vi "AnalyzerDataToString.vi"(8 "ErrorIn":errorcluster, 11 "WebServicesData":T2) -> (0 "ErrorOut":errorcluster, 3 "String":string)   [LabVIEW 2019]
uses:
  MobileAnalyzer/mainVIs/communicateWebServicesVIs/WebServicesData.ctl
  MobileAnalyzer/mainVIs/analyzeAccelerationDataVIs/AccelerationDataFrames.ctl
  MobileAnalyzer/mainVIs/UIVIs/UIOutput.ctl
  <vilib>/wsapi/NI_WebServices.lvlib
panel:
  in  "VisualizedData":enum32{"Page 1", "Page 2"}(tab)
  out "Phases":T1(graph)
  out "Amplitudes":cluster{"f0":dbl, "df":dbl, "real part":dbl[]}[](graph)
  out "Acceleration":waveform(dbl)[](graph)
  out "Aquiring data":bool
  out "FIFO overflow":bool
  out "Analyzing data":bool
  out "AnalyzerError":errorcluster
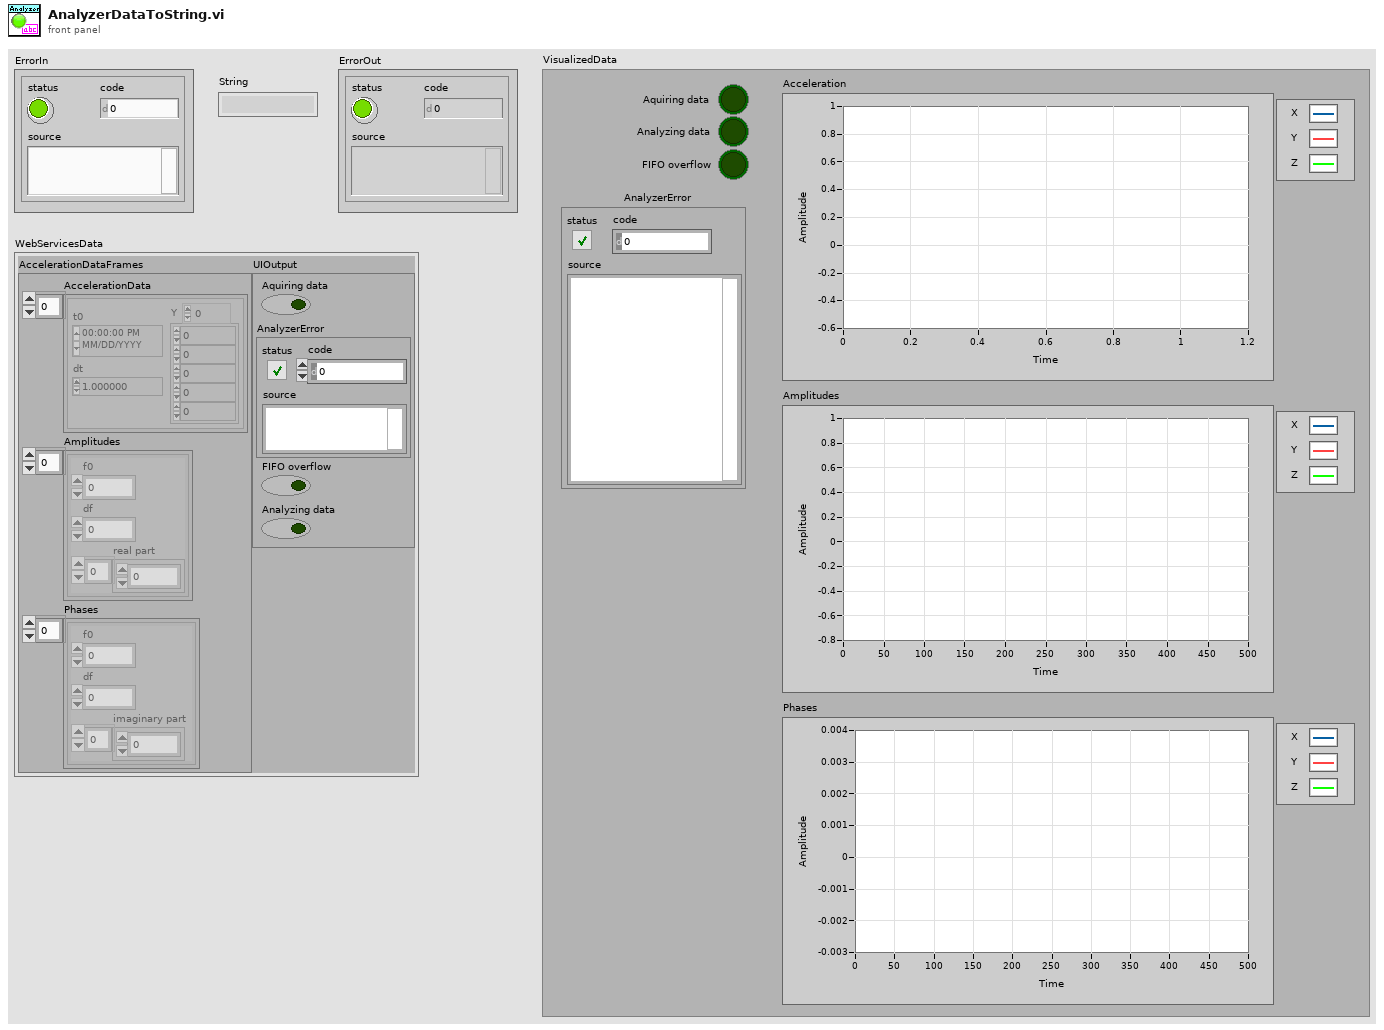
[diagram p1: front panel]
types:
  T1 = cluster{"f0":dbl, "df":dbl, "imaginary part":dbl[]}[]
  T2 = typedef "WebServicesData.ctl" = cluster{"AccelerationDataFrames":T3, "UIOutput":T4}
  T3 = typedef "AccelerationDataFrames.ctl" = cluster{"AccelerationData":waveform(dbl)[], "Amplitudes":cluster{"f0":dbl, "df":dbl, "real part":dbl[]}[], "Phases":cluster{"f0":dbl, "df":dbl, "imaginary part":dbl[]}[]}
  T4 = typedef "UIOutput.ctl" = cluster{"Aquiring data":bool, "AnalyzerError":errorcluster, "FIFO overflow":bool, "Analyzing data":bool}
  T5 = typedef "imagedata.ctl" = cluster{"image type":i32, "image depth":i32, "image":u8[], "mask":u8[], "colors":u32[], "Rectangle":cluster{"left":i16, "top":i16, "right":i16, "bottom":i16}}
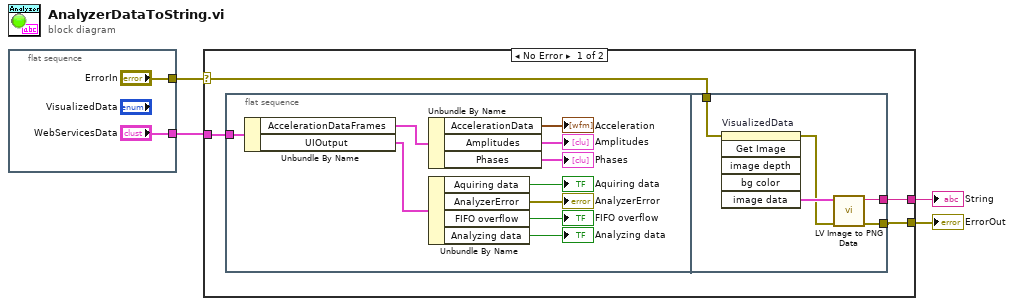
[diagram p0: block diagram]
diagram:
  n1 = flat-sequence {
    tunnel: ["WebServicesData"] -> w3
    tunnel: ["ErrorIn"] -> w2
    frame #0 {
    }
  }
  n2 = case shown="No Error" w2 {
    selector: w2 -> [w9 w26]
    tunnel: w3 -> [w10 _]
    tunnel: [w8 w26] -> w4
    tunnel: [w7 _] -> w1
    frame No Error {
      n3 = flat-sequence {
        tunnel: w10 -> [w20]
        tunnel: w9 -> [w25]
        tunnel: [w21] -> w8
        tunnel: [w22] -> w7
        frame #0 {
          n4 = Unbundle By Name(w20) -> ("AccelerationDataFrames"=w19:T3, "UIOutput"=w15:T4)
          n5 = Unbundle By Name(w19) -> ("AccelerationData"=→"Acceleration":waveform(dbl)[], "Amplitudes"=→"Amplitudes":cluster{"f0":dbl, "df":dbl, "real part":dbl[]}[], "Phases"=→"Phases":T1)
          n6 = Unbundle By Name(w15) -> ("Aquiring data"=→"Aquiring data":bool, "AnalyzerError"=→"AnalyzerError":errorcluster, "FIFO overflow"=→"FIFO overflow":bool, "Analyzing data"=→"Analyzing data":bool)
        }
        frame #1 {
          n7 = invoke on="VisualizedData" class="TabCtl (strict)" method="Get Image"(error in=w25) -> (error out=w23:errorcluster, "image data"=w24:T5)  [unwired: 5 in, 4 out]
          n8 = call <vilib>:"LV Image to PNG Data.vi"("error in (no error)"=w23, "image data"=w24) -> ("error out"=w21:errorcluster, "png data"=w22:string)  [unwired: 8 in]
        }
      }
    }
    frame Error {
    }
  }
  "String" <- w1
  "ErrorOut" <- w4
